vi "4461 Calibrate Phase.vi"(8 "error in (no error)":errorcluster, 9 "Boolean":bool, 10 "Results":T1 {"Results (Dictionary)"."value" format="%#_6p"}, 11 "Instrument.DAQ in":refnum<class "Instrument.DAQ.lvclass">) -> (0 "error out":errorcluster, 3 "Instrument.DAQ out":refnum<class "Instrument.DAQ.lvclass">)   [LabVIEW 2019, in "Instrument.DAQ.lvclass"]
uses:
  Instrument.DAQ.lvclass
  Typedefs/Results--Cluster.ctl
  Instrument.Lockin/Typedefs/Results Type--Enum.ctl
  Instrument.DAQ.lvclass/Instrument.DAQ.ctl
  Instrument.Lockin/Instrument.Lockin.lvclass
  <vilib>/addons/control/pid/NI_PID_pid.lvlib
  <vilib>/addons/control/pid/pid.llb/PID Control Input Filter (DBL).vi
panel:
  in  "Map":cluster{"output":i32, "input":i32}[](array[cluster])
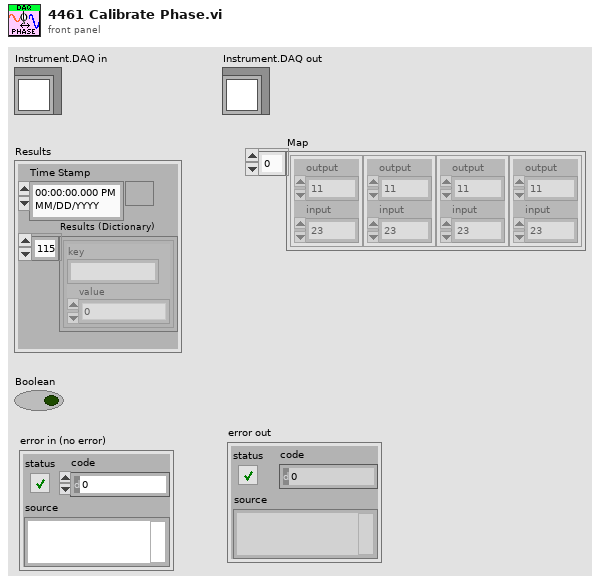
[diagram p1: front panel]
types:
  T1 = typedef "Instrument.DAQ.lvclass/Results--Cluster.ctl" = cluster{"Time Stamp":timestamp, "Results (Dictionary)":cluster{"key":string, "value":dbl}[]}
  T2 = typedef "Instrument.Lockin.lvclass/Results Type--Enum.ctl" = enum16{"X", "Y", "R", "Theta", "Mean"}
  T3 = typedef "Instrument.DAQ.lvclass/AO.Channel--Cluster--Array.ctl" = T4[]
  T4 = typedef "Instrument.DAQ.lvclass/AO.Channel--Cluster.ctl" = cluster{"Enable?":bool, "Channel":i32, "Amplitude":dbl, "Offset":dbl, "Frequency":dbl, "Phase":dbl, "Function":T5, "Sweeping?":bool}
  T5 = typedef "Instrument.DAQ.lvclass/AO.Channel.Function--Enum.ctl" = enum16{"Sine", "Triangle", "Square"}
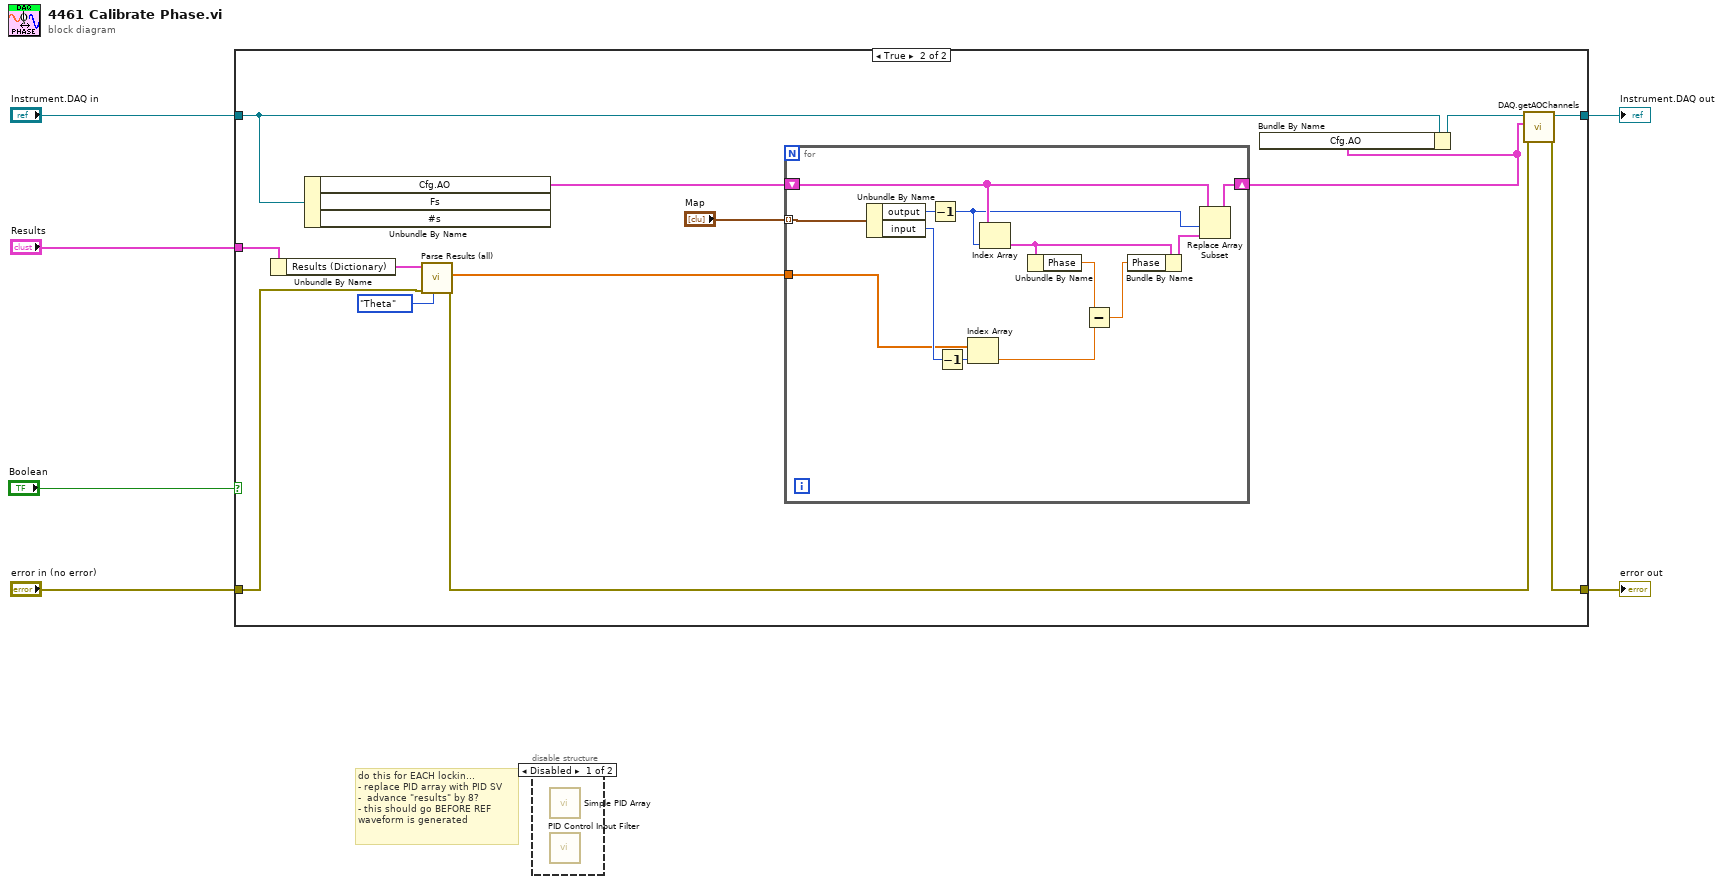
[diagram p0: block diagram]
diagram:
  # "do this for EACH lockin...\n- replace PID array with PID SV\n-  advance \"results\" by 8?\n- this should go BEFORE REF\nwaveform is generated"
  n1 = case shown="True" "Boolean" {
    tunnel: "Instrument.DAQ in" -> [w8 w21]
    tunnel: "Results" -> [_ w20]
    tunnel: "error in (no error)" -> [w7 w19]
    tunnel: [w8 w18] -> w3
    tunnel: [w7 w10] -> w2
    frame False {
    }
    frame True {
      n2 = Unbundle By Name(w20) -> ("Results (Dictionary)"=w17:cluster{"key":string, "value":dbl}[])
      n3 = Unbundle By Name(w21) -> ("Cfg.AO"=w13:T3)  [unwired: 2 out]
      n4 = call "Parse Results (all).vi"("Type"=Results_Type--Enum."Theta", "error in (no error)"=w19, "Results (Dictionary)"=w17) -> ("error out"=w14:errorcluster, "Data"=w9:dbl[])  [unwired: 5 in, 2 out]
      n5 = for {
        tunnel: "Map" -> [w31] mode=indexing
        shift-right: [w26] -> w11
        shift-left: w13 -> [w33]
        tunnel: w9 -> [w25]
        n6 = Unbundle By Name(w31) -> ("output"=w30:i32, "input"=w29:i32)
        n7 = Decrement(x=w30) -> (x-1=w27:i32)
        n8 = Decrement(x=w29) -> (x-1=w28:i32)
        n9 = Index Array(array=w25, index=w28) -> (element=w23:dbl)
        n10 = Index Array(array=w33, index=w27) -> (element=w34:T4)
        n11 = Unbundle By Name(w34) -> ("Phase"=w24:dbl)
        n12 = Subtract(x=w24, y=w23) -> (x-y=w22:dbl)
        n13 = Bundle By Name(cluster=w34, "Phase"=w22) -> (w32:T4)
        n14 = Replace Array Subset(array=w33, new element=w32, index=w27) -> (w26:T3)
      }
      n15 = Bundle By Name(cluster=w21, "Cfg.AO"=w11) -> (w15:refnum<class "Instrument.DAQ.lvclass">)
      n16 = call "DAQ.getAOChannels.vi"("error in (no error)"=w14, "Channels: AO"=w11, "Instrument.DAQ"=w15) -> ("error out"=w10:errorcluster, "Instrument.DAQ out"=w18:refnum<class "Instrument.DAQ.lvclass">)  [unwired: 7 in]
    }
  }
  "Instrument.DAQ out" <- w3
  "error out" <- w2
  n17 = disable-structure shown="Disabled" {
    frame Disabled {
      n18 = call "Simple PID Array.vi"() -> ()  [unwired: 11 in, 1 out]
      n19 = call-poly <vilib>:"PID Control Input Filter.vi"() -> ()  [unwired: 5 in, 1 out]
    }
    frame Enabled {
    }
  }
